vi "Test_GetTime.vi"() -> ()   [LabVIEW 2018]
uses:
  C:/Viviota/Projects/R&D/LabVIEW_ORM/source/libraries/kdb/KpNet.KdbPlusClient.dll
  libraries/kdb/KpNet.KdbPlusClient.dll
  System.Data
panel:
  out "data":u8[](array[numeric])
  out "ToString 2":string
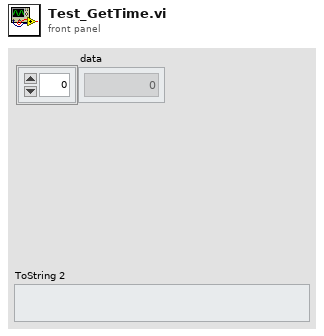
[diagram p1: front panel]
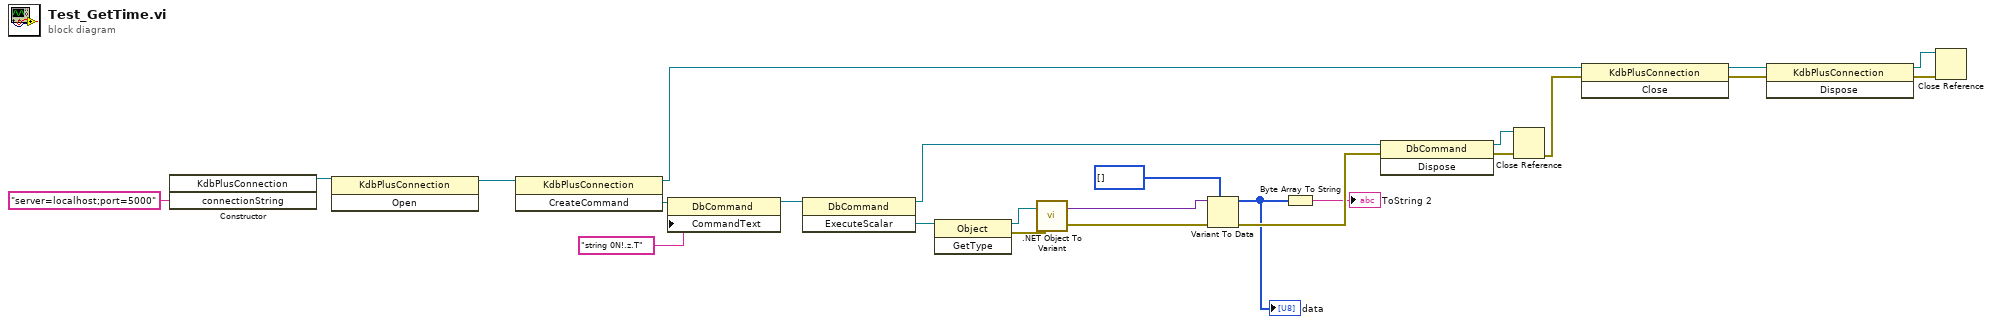
[diagram p0: block diagram]
diagram:
  n1 = constructor class="KdbPlusConnection"("connectionString"="server=localhost;port=5000") -> (reference out=w23:refnum<k24>)  [unwired: 3 in, 3 out]
  n2 = invoke class="KdbPlusConnection" method="Open"(reference=w23) -> (reference out=w22:refnum<k24>)  [unwired: 2 in, 2 out]
  n3 = invoke class="KdbPlusConnection" method="CreateCommand"(reference=w22) -> (reference out=w17:refnum<k24>, "CreateCommand"=w21:refnum<k24>)  [unwired: 2 in, 1 out]
  n4 = property class="DbCommand"(reference=w21, "CommandText"="string 0N!.z.T") -> (reference out=w19:refnum<k24>)  [unwired: 1 in, 1 out]
  n5 = invoke class="DbCommand" method="ExecuteScalar"(reference=w19) -> (reference out=w18:refnum<k24>, "ExecuteScalar"=w9:refnum<k24>)  [unwired: 2 in, 1 out]
  n6 = invoke class="Object" method="GetType"(reference=w9) -> (reference out=w8:refnum<k24>, error out=w7:errorcluster)  [unwired: 2 in, 1 out]
  n7 = call <vilib>:".NET Object To Variant.vi"("error in (no error)"=w7, ".NET object"=w8) -> ("error out"=w6:errorcluster, "variant"=w4:variant)
  n8 = Variant To Data(error in=w6, type=u8[] [], Variant=w4) -> (data=w2:u8[], error out=w5:errorcluster)
  "data" <- w2
  n9 = Byte Array To String(unsigned byte array=w2) -> (string=→"ToString 2":string)
  n10 = invoke class="DbCommand" method="Dispose"(reference=w18, error in=w5) -> (reference out=w14:refnum<k24>, error out=w15:errorcluster)  [unwired: 1 in, 1 out]
  n11 = Close Reference(reference=w14, error in (no error)=w15) -> (error out=w10:errorcluster)
  n12 = invoke class="KdbPlusConnection" method="Close"(reference=w17, error in=w10) -> (reference out=w16:refnum<k24>, error out=w11:errorcluster)  [unwired: 1 in, 1 out]
  n13 = invoke class="KdbPlusConnection" method="Dispose"(reference=w16, error in=w11) -> (reference out=w12:refnum<k24>, error out=w13:errorcluster)  [unwired: 1 in, 1 out]
  n14 = Close Reference(reference=w12, error in (no error)=w13) -> ()  [unwired: 1 out]
